vi "Add Fruit.vi"(8 "error in (no error)":errorcluster, 11 "Board_Game in":refnum<class "Board_Game.lvclass">) -> (0 "error out":errorcluster, 3 "Board_Game out":refnum<class "Board_Game.lvclass">)   [LabVIEW 2021, in "Board_Game.lvclass"]
uses:
  Board_Game.lvclass
  Board_Game.lvclass/Board_Game.ctl
  <vilib>/numeric/Random Number (Range) I64.vi
  <vilib>/numeric/sub_Random U32.vi
  SnakeGame/Snake.lvclass
  Fruit/Fruit.lvclass
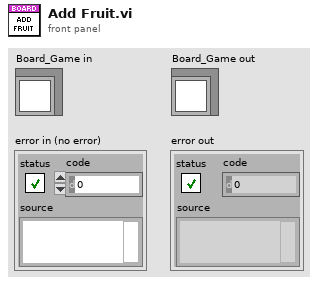
[diagram p1: front panel]
types:
  T1 = typedef "Position.ctl" = cluster{"X":u32, "Y":u32}
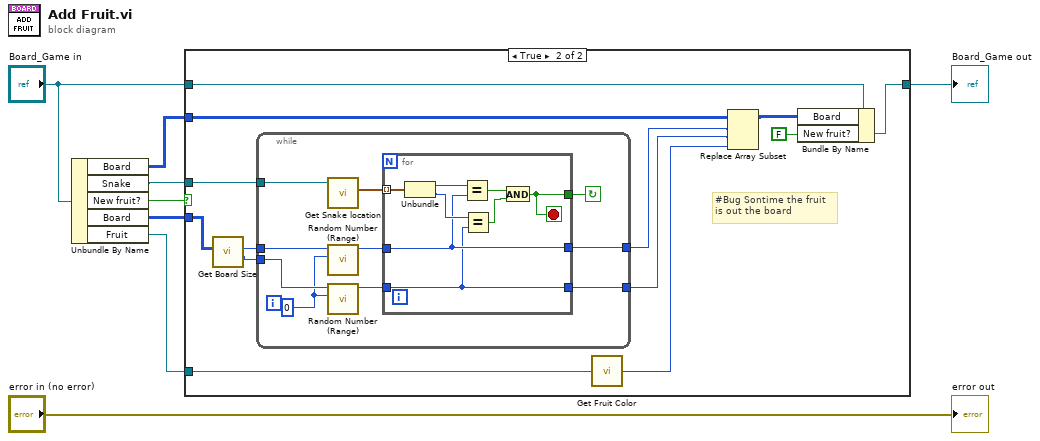
[diagram p0: block diagram]
diagram:
  n1 = Unbundle By Name("Board_Game in") -> ("Board"=w2:u32[][], "Snake"=w3:refnum<class "Snake.lvclass">, "New fruit?"=w7:bool, "Board"=w4:u32[][], "Fruit"=w1:refnum<class "Fruit.lvclass">)
  n2 = case shown="True" w7 {
    tunnel: "Board_Game in" -> [w9 w22]
    tunnel: [w9 w21] -> w5
    tunnel: w4 -> [_ w19]
    tunnel: w3 -> [_ w16]
    tunnel: w2 -> [_ w15]
    tunnel: w1 -> [_ w10]
    frame False {
    }
    frame True {
      # "#Bug Sontime the fruit\nis out the board"
      n3 = call "Get Board Size.vi"("Board"=w19) -> ("Y"=w17:i32, "X"=w18:i32)  [unwired: 9 in]
      n4 = while {
        tunnel: w18 -> [w32]
        tunnel: w17 -> [w31]
        tunnel: w16 -> [w29]
        tunnel: [w24] -> w13
        tunnel: [w23] -> w12
        stop <- w25 continue-if-true
        w30 = i64 0 ("lower bound (-100)")
        n5 = call-dynamic "Get Snake location.vi"("Snake in"=w29) -> ("Snake location"=w28:T1[])  [unwired: 8 in, 2 out]
        n6 = call-poly <vilib>:"Random Number (Range).vi"("lower bound (-100)"=w30, "upper bound (100)"=w32) -> ("number"=w27:i64)  [unwired: 9 in]
        n7 = call-poly <vilib>:"Random Number (Range).vi"("lower bound (-100)"=w30, "upper bound (100)"=w31) -> ("number"=w26:i64)  [unwired: 9 in]
        n8 = for {
          tunnel: w28 -> [w40] mode=indexing
          tunnel: w27 -> [w34]
          tunnel: w26 -> [w33]
          tunnel: [w35] -> w25
          tunnel: [w34] -> w24
          tunnel: [w33] -> w23
          stop <- w35 stop-if-true
          n9 = Unbundle(w40) -> ("X"=w39:u32, "Y"=w38:u32)
          n10 = Equal?(x=w39, y=w34) -> (x = y?=w37:bool)
          n11 = Equal?(x=w38, y=w33) -> (x = y?=w36:bool)
          n12 = And(x=w37, y=w36) -> (x .and. y?=w35:bool)
        }
      }
      n13 = call "Get Fruit Color.vi"("Fruit in"=w10) -> ("FruitColor"=w11:u32)  [unwired: 8 in]
      n14 = Replace Array Subset(array=w15, new element=w11, index (row)=w13, index (col)=w12) -> (w14:u32[][])
      n15 = Bundle By Name(cluster=w22, "Board"=w14, "New fruit?"=FALSE) -> (w21:refnum<class "Board_Game.lvclass">)
    }
  }
  "Board_Game out" <- w5
  "error out" <- "error in (no error)"
